vi "Wybierz przebiegi.vi"(7 "Mode":u32, 8 "Wybierz drugi monitorowanyprzebieg":i32, 9 "Wybierz pierwszy monitorowanyprzebieg":i32, 11 "Wybierz monitorowany przebieg":i32) -> (1 "WPlots":i32[](array[numeric]), 3 "Plot":i32)   [LabVIEW 2013]
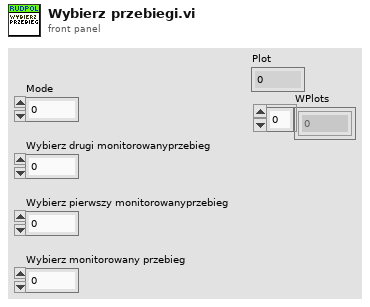
[diagram p1: front panel]
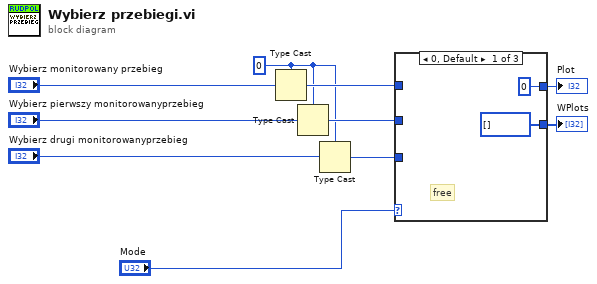
[diagram p0: block diagram]
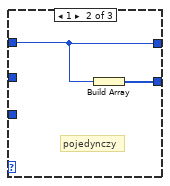
[diagram p2: hidden frame]
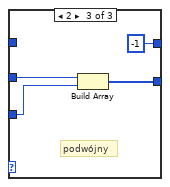
[diagram p3: hidden frame]
diagram:
  w6 = 0
  n1 = Type Cast(type=w6, x="Wybierz monitorowany przebieg") -> (*(type *) &x=w8:i32)
  n2 = Type Cast(type=w6, x="Wybierz pierwszy monitorowanyprzebieg") -> (*(type *) &x=w9:i32)
  n3 = Type Cast(type=w6, x="Wybierz drugi monitorowanyprzebieg") -> (*(type *) &x=w10:i32)
  n4 = case shown="0, Default" "Mode" {
    tunnel: w8 -> [_ w13 _]
    tunnel: w9 -> [_ _ w18]
    tunnel: w10 -> [_ _ w17]
    tunnel: [0 w13 -1] -> w2
    tunnel: [i32[] [] w14 w16] -> w1
    frame 0, Default {
      # "free"
    }
    frame 1 {
      # "pojedynczy"
      n5 = Build Array(w13) -> (w14:i32[])
    }
    frame 2 {
      # "podwójny"
      n6 = Build Array(w18, w17) -> (w16:i32[])
    }
  }
  "Plot" <- w2
  "WPlots" <- w1
